vi "Comparator.vi"(1 "Current Location":T1 {"Shooter Throttle" min=-360.0 max=360.0}, 2 "Target Location":T1 {"Shooter Throttle" min=-360.0 max=360.0}, 3 "Rotate Tolerance":dbl, 4 "Strafe Tolerance":dbl) -> (0 "In range?":bool)   [LabVIEW 2023]
doc: "Checks the robot's current position and determines if it is within the tolerances defined by the setpoint. When x, y, and yaw are within range, this function will return \"true\"."
uses:
  Variables and Definitions/DB Auton Data.ctl
panel:
  # "Takes precedence\nfrom Tol"
  # "Takes precedence\nfrom Tol"
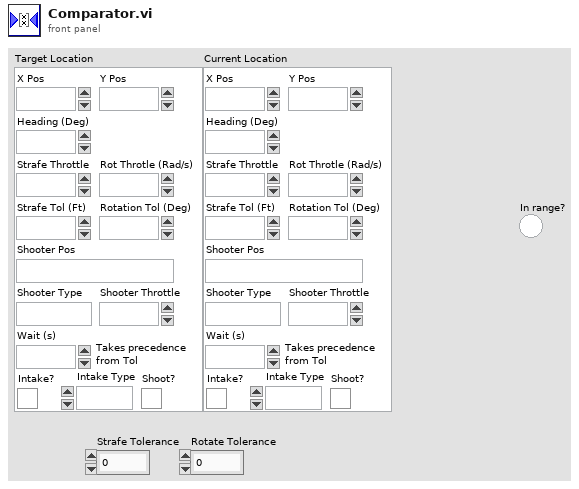
[diagram p1: front panel]
types:
  T1 = typedef "DB Auton Data.ctl" = cluster{"X Pos":dbl, "Y Pos":dbl, "Heading (Deg)":dbl, "Strafe Throttle":dbl, "Rot Throtle (Rad/s)":dbl, "Strafe Tol (Ft)":dbl, "Rotation Tol (Deg)":dbl, "Shooter Pos":enum16{"Travel", "Speaker", "Amp"}, "Intake Type":enum16{"Front", "Center"}, "Intake?":bool, "Shooter Type":enum16{"Manual", "Automatic"}, "Shooter Throttle":dbl, "Wait (s)":dbl, "Shoot?":bool}
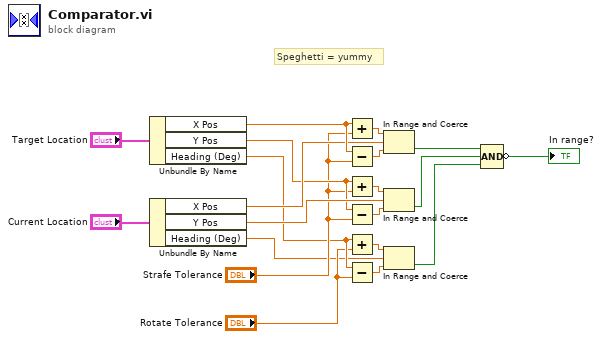
[diagram p0: block diagram]
diagram:
  # "Speghetti = yummy"
  n1 = Unbundle By Name("Target Location") -> ("X Pos"=w18:dbl, "Y Pos"=w13:dbl, "Heading (Deg)"=w9:dbl)
  n2 = Unbundle By Name("Current Location") -> ("X Pos"=w17:dbl, "Y Pos"=w14:dbl, "Heading (Deg)"=w3:dbl)
  n3 = Add(x=w18, y="Strafe Tolerance") -> (x+y=w19:dbl)
  n4 = Subtract(x=w18, y="Strafe Tolerance") -> (x-y=w20:dbl)
  n5 = Add(x=w13, y="Strafe Tolerance") -> (x+y=w15:dbl)
  n6 = Subtract(x=w13, y="Strafe Tolerance") -> (x-y=w16:dbl)
  n7 = Add(x=w9, y="Rotate Tolerance") -> (x+y=w11:dbl)
  n8 = Subtract(x=w9, y="Rotate Tolerance") -> (x-y=w10:dbl)
  n9 = In Range and Coerce(upper limit=w19, x=w17, lower limit=w20) -> (In Range?=w7:bool)  [unwired: 1 out]
  n10 = In Range and Coerce(upper limit=w15, x=w14, lower limit=w16) -> (In Range?=w6:bool)  [unwired: 1 out]
  n11 = In Range and Coerce(upper limit=w11, x=w3, lower limit=w10) -> (In Range?=w5:bool)  [unwired: 1 out]
  n12 = Compound Arithmetic op=AND(w7, w6, w5) -> (invert →"In range?":bool)
